vi "Joystick to Dashboard.vi"(8 "Raw Buttons":T1, 9 "Raw Axes":T2, 11 "refnum name":string) -> ()   [LabVIEW 2014]
doc: "Sends values from the joystick to the dashboard."
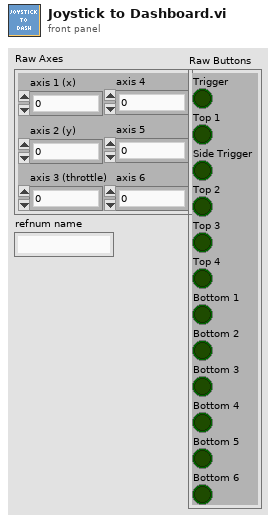
[diagram p1: front panel]
types:
  T1 = cluster{"Trigger":bool, "Top 1":bool, "Side Trigger":bool, "Top 2":bool, "Top 3":bool, "Top 4":bool, "Bottom 1":bool, "Bottom 2":bool, "Bottom 3":bool, "Bottom 4":bool, "Bottom 5":bool, "Bottom 6":bool}
  T2 = cluster{"axis 1 (x)":dbl, "axis 2 (y)":dbl, "axis 3 (throttle)":dbl, "axis 4":dbl, "axis 5":dbl, "axis 6":dbl}
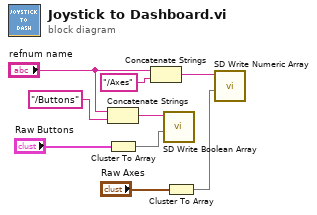
[diagram p0: block diagram]
diagram:
  n1 = Concatenate Strings("refnum name", "/Buttons" ("Name")) -> (w2:string)
  n2 = Cluster To Array(cluster="Raw Buttons") -> (array=w9:bool[])
  n3 = Concatenate Strings("refnum name", "/Axes" ("Name")) -> (w4:string)
  n4 = call <vilib>:"SD Write Boolean Array.vi"("Boolean Array"=w9, "Name"=w2) -> ()  [unwired: 8 in, 2 out]
  n5 = Cluster To Array(cluster="Raw Axes") -> (array=w8:dbl[])
  n6 = call <vilib>:"SD Write Numeric Array.vi"("Numeric Array"=w8, "Name"=w4) -> ()  [unwired: 8 in, 2 out]
